vi "SendPluginDeactivatedEvent.vi"(8 "error in (no error)":errorcluster, 11 "_LVCMPlugin in":refnum<class "GCMPlugin.lvclass">) -> (0 "error out":errorcluster, 3 "_LVCMPlugin out":refnum<class "GCMPlugin.lvclass">)   [LabVIEW 2014, in "GCMPlugin.lvclass"]
uses:
  GCMPlugin/GCMPlugin.lvclass
  GCMPlugin/GCMPlugin.lvclass/GCMPlugin.ctl
  <vilib>/event_ctls.llb/usereventprio.ctl
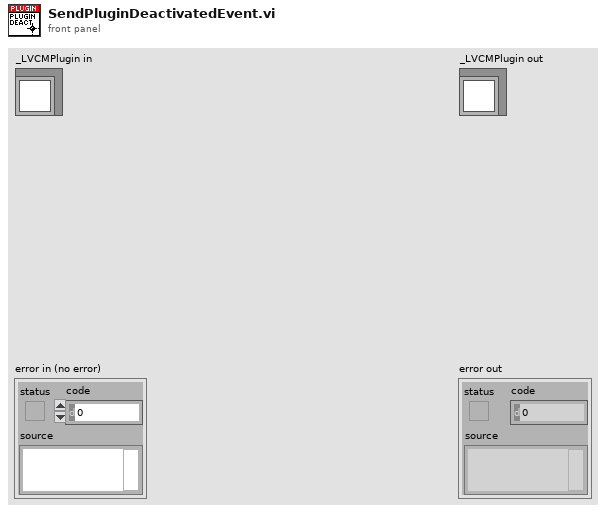
[diagram p1: front panel]
types:
  T1 = typedef "usereventprio.ctl" = enum32{"high priority", "normal priority"}
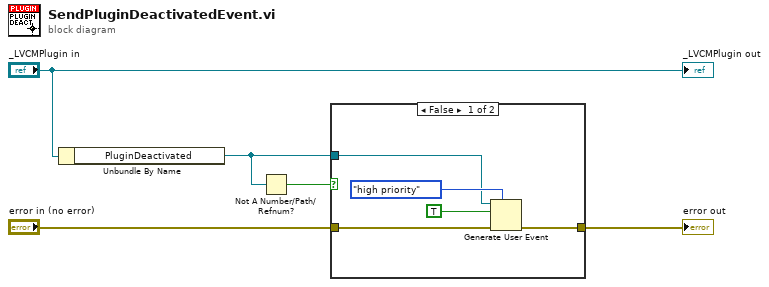
[diagram p0: block diagram]
diagram:
  n1 = Unbundle By Name("_LVCMPlugin in") -> ("PluginDeactivated"=w2:refnum<user-event>)
  n2 = Not A Number/Path/Refnum?(number/path/refnum=w2) -> (NaN/Path/Refnum?=w1:bool)
  n3 = case shown="False" w1 {
    tunnel: "error in (no error)" -> [w10 w11]
    tunnel: [w9 w11] -> w4
    tunnel: w2 -> [w6 _]
    frame False {
      n4 = Generate User Event(priority (normal)=usereventprio."high priority", user event=w6, event data cluster=TRUE ("event data"), error in=w10) -> (error out=w9:errorcluster)  [unwired: 1 out]
    }
    frame True {
    }
  }
  "error out" <- w4
  "_LVCMPlugin out" <- "_LVCMPlugin in"
